vi "Get Config.vi"() -> (3 "Database Record":T1={"Door Open"=1.0, "Travel Time"=1.0, "Door Close"=1.0, "Inactivity Time"=1.0} {"Inactivity Time" format="%#_g Seconds"; "Door Close" format="%#_g Seconds"; "Travel Time" format="%#_g Seconds"; "Door Open" format="%#_g Seconds"})   [LabVIEW 2020, in "Configuration Database.lvlib"]
doc: "Interface to obtain databasare resourcese / records.\n[Covers: CD2] \n[Covers: CD4]"
uses:
  Configuration Database.lvlib
  Controls/DB Record.ctl
  Controls/FGV Mode.ctl
panel:
  out "error out":errorcluster
  in  "error in":errorcluster
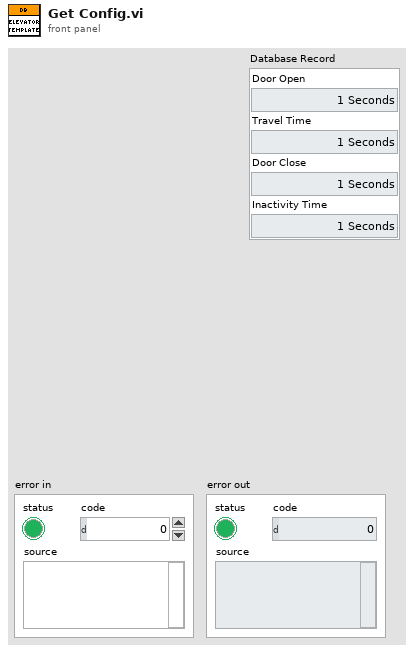
[diagram p1: front panel]
types:
  T1 = typedef "Configuration Database.lvlib/DB Record.ctl" = cluster{"Door Open":dbl, "Travel Time":dbl, "Door Close":dbl, "Inactivity Time":dbl}
  T2 = typedef "Configuration Database.lvlib/FGV Mode.ctl" = enum16{"Initialize", "Get", "Update", "Close"}
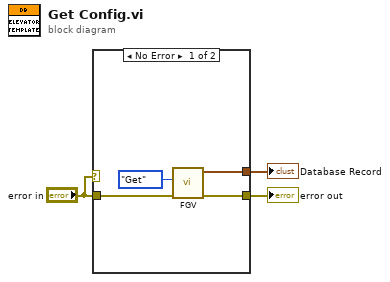
[diagram p0: block diagram]
diagram:
  n1 = case shown="No Error" "error in" {
    tunnel: [w5 w8] -> w3
    tunnel: "error in" -> [w6 w8]
    tunnel: [w7 _] -> w1
    frame No Error {
      n2 = call "FGV.vi"("error in"=w6, "Mode"=FGV_Mode."Get") -> ("error out"=w5:errorcluster, "Database Record"=w7:T1)  [unwired: 8 in]
    }
    frame Error {
    }
  }
  "error out" <- w3
  "Database Record" <- w1
